vi "CheckCamIP.vi"(11 "address in":string) -> (3 "address out":string)   [LabVIEW 2020]
uses:
  <vilib>/Utility/config.llb/NI_LVConfig.lvlib
  <vilib>/Utility/config.llb/Read Key (String).vi
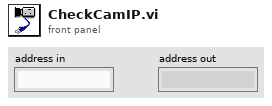
[diagram p1: front panel]
types:
  T1 = typedef "NI_LVConfig.lvlib/Config Data RefNum.ctl" = refnum<k1>
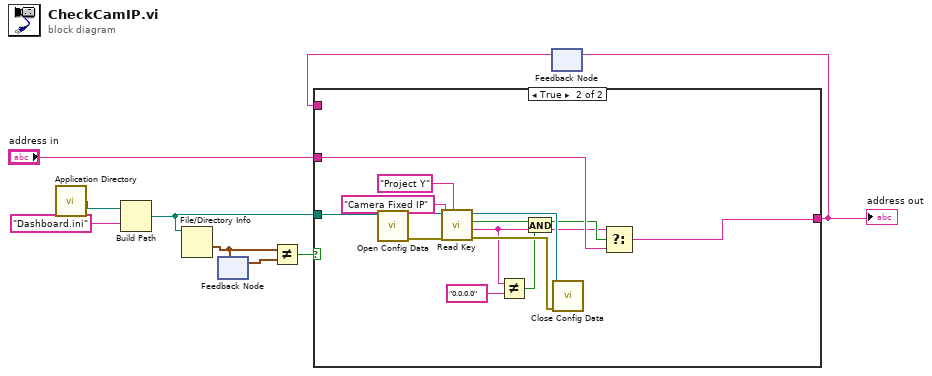
[diagram p0: block diagram]
diagram:
  n1 = call <vilib>:"Application Directory.vi"() -> ("Application Directory"=w9:path)
  n2 = Build Path(base path=w9, name or relative path="Dashboard.ini") -> (appended path=w7:path)
  n3 = File/Directory Info(path=w7) -> (last mod=w6:timestamp)  [unwired: 1 in, 6 out]
  n4 = feedback-in #1(w6) -> ()
  n5 = feedback #1() -> (w5:timestamp)  [unwired: 1 in]
  n6 = Not Equal?(x=w6, y=w5) -> (x != y?=w4:bool)
  n7 = feedback #2() -> (w2:string)  [unwired: 1 in]
  n8 = case shown="True" w4 {
    tunnel: w7 -> [_ w24]
    tunnel: "address in" -> [_ w19]
    tunnel: [w10 w18] -> w1
    tunnel: w2 -> [w10 _]
    frame False {
    }
    frame True {
      n9 = call <vilib>:"Open Config Data.vi"("configuration file path"=w24) -> ("error out"=w22:errorcluster, "refnum"=w23:T1)  [unwired: 8 in, 1 out]
      n10 = call-poly <vilib>:"Read Key.vi"("section"="Project Y", "error in (no error)"=w22, "key"="Camera Fixed IP", "refnum"=w23) -> ("error out"=w17:errorcluster, "value"=w13:string, "found?"=w16:bool, "refnum out"=w15:T1)  [unwired: 4 in]
      n11 = Not Equal?(x=w13, y="0.0.0.0") -> (x != y?=w12:bool)
      n12 = And(x=w16, y=w12) -> (x .and. y?=w14:bool)
      n13 = call <vilib>:"Close Config Data.vi"("error in (no error)"=w17, "refnum"=w15) -> ()  [unwired: 8 in, 2 out]
      n14 = Select(t=w13, s=w14, f=w19) -> (s? t:f=w18:string)
    }
  }
  "address out" <- w1
  n15 = feedback-in #2(w1) -> ()
